vi "Cholesky Factorization Rank-1 Update_Givens Rotation Update (DBL).vi"(8 "Y In":dbl[](array[numeric]), 9 "X In":dbl[](array[numeric]), 10 "b":dbl, 11 "a":dbl) -> (1 "Y Out":dbl[](array[numeric]), 2 "X Out":dbl[](array[numeric]), 3 "v":dbl)   [LabVIEW 2020, in "NI_AAL_LinAlg.lvlib"]
uses:
  <vilib>/Analysis/NI_AAL_LinAlg.lvlib
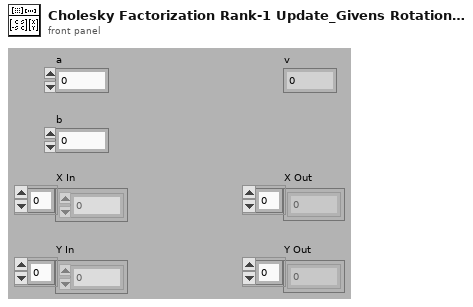
[diagram p1: front panel]
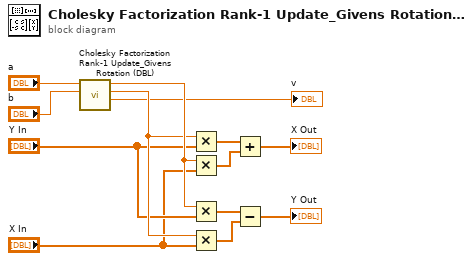
[diagram p0: block diagram]
diagram:
  n1 = call <vilib>:"Cholesky Factorization Rank-1 Update_Givens Rotation (DBL).vi"("b"="b", "a"="a") -> ("v"=→"v":dbl, "s"=w8:dbl, "c"=w9:dbl)  [unwired: 7 in]
  n2 = Multiply(x=w8, y="Y In") -> (x*y=w10:dbl[])
  n3 = Multiply(x=w9, y="X In") -> (x*y=w11:dbl[])
  n4 = Multiply(x=w9, y="Y In") -> (x*y=w13:dbl[])
  n5 = Multiply(x=w8, y="X In") -> (x*y=w12:dbl[])
  n6 = Add(x=w10, y=w11) -> (x+y=→"X Out":dbl[])
  n7 = Subtract(x=w13, y=w12) -> (x-y=→"Y Out":dbl[])
